vi "Fetch Class Parents Info.vi"(8 "error in (no error)":errorcluster, 11 "LVClassLibrary in":refnum<vi>) -> (0 "error out":errorcluster, 1 "Parent Interfaces":refnum<vi>[](array[refnum]), 2 "Parent Class Info":T1[](array[typedef]), 3 "LVClassLibrary out":refnum<vi>)   [LabVIEW 2023, in "VIDoc Parsing.lvlib"]
uses:
  VIDoc Parsing.lvlib
  TypeDefs/Base Class Info Cluster.ctl
  <vilib>/picture/picture.llb/imagedata.ctl
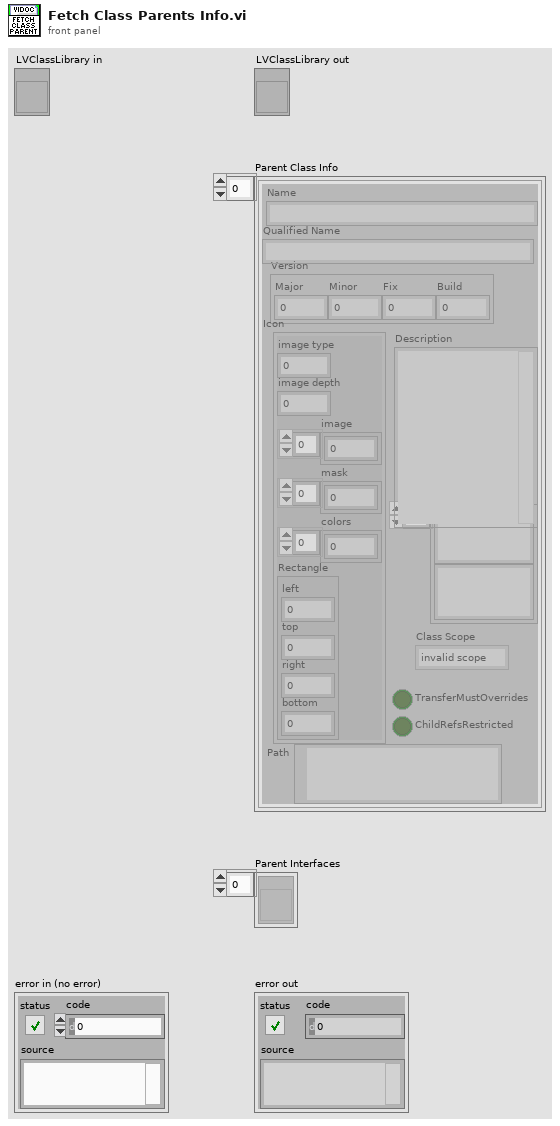
[diagram p1: front panel]
types:
  T1 = typedef "VIDoc Parsing.lvlib/Base Class Info Cluster.ctl" = cluster{"Name":string, "Icon":T2, "Version":cluster{"Major":u16, "Minor":u16, "Fix":u16, "Build":u16}, "Description":string, "Friends":string[], "ChildRefsRestricted":bool, "TransferMustOverrides":bool, "Path":path, "Qualified Name":string, "Class Scope":enum32{"invalid scope", "public", "private", "protected", "community"}}
  T2 = typedef "imagedata.ctl" = cluster{"image type":i32, "image depth":i32, "image":u8[], "mask":u8[], "colors":u32[], "Rectangle":cluster{"left":i16, "top":i16, "right":i16, "bottom":i16}}
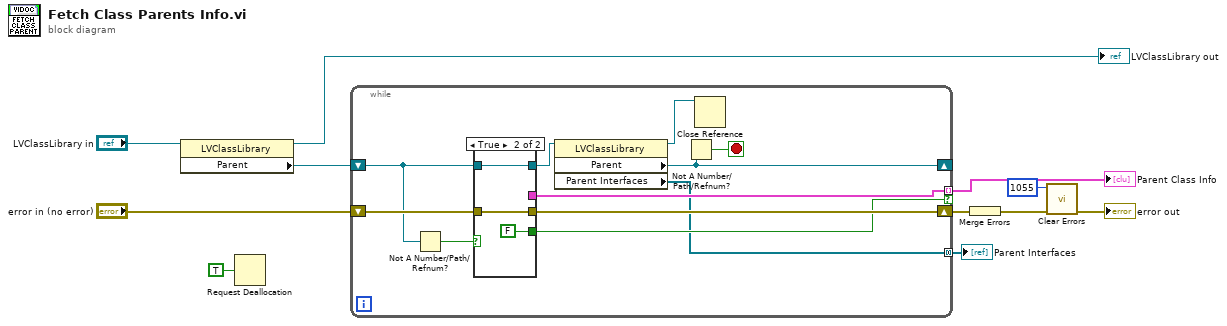
[diagram p0: block diagram]
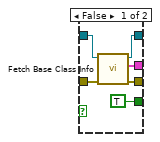
[diagram p2: hidden frame]
diagram:
  n1 = property class="LVClassLibrary"(reference="LVClassLibrary in") -> (reference out=→"LVClassLibrary out":refnum<vi>, "Parent"=w2:refnum<vi>)  [unwired: 1 in, 1 out]
  n2 = Request Deallocation(TRUE ("flag")) -> ()
  n3 = while {
    shift-right: [w18] -> _
    shift-left: w2 -> [w16]
    tunnel: [w17] -> w8 mode=indexing if=w14
    shift-right: [w20] -> w9
    shift-left: "error in (no error)" -> [w21]
    tunnel: [w13] -> w3 mode=concatenating
    stop <- w22 stop-if-true
    n4 = Not A Number/Path/Refnum?(number/path/refnum=w16) -> (NaN/Path/Refnum?=w15:bool)
    n5 = case shown="True" w15 {
      tunnel: w21 -> [w28 w30]
      tunnel: [w27 w30] -> w20
      tunnel: [w26 w31] -> w19
      tunnel: [w25 _] -> w17
      tunnel: w16 -> [w24 w31]
      tunnel: [TRUE FALSE] -> w14
      frame False {
        n6 = call "Fetch Base Class Info.vi"("error in (no error)"=w28, "LVClassLibrary in"=w24) -> ("error out"=w27:errorcluster, "Base Class Info"=w25:T1, "LVClassLibrary out"=w26:refnum<vi>)  [unwired: 7 in]
      }
      frame True {
      }
    }
    n7 = property class="LVClassLibrary"(reference=w19) -> (reference out=w12:refnum<vi>, "Parent"=w18:refnum<vi>, "Parent Interfaces"=w13:refnum<vi>[])  [unwired: 1 in, 1 out]
    n8 = Not A Number/Path/Refnum?(number/path/refnum=w18) -> (NaN/Path/Refnum?=w22:bool)
    n9 = Close Reference(reference=w12) -> ()  [unwired: 1 in, 1 out]
  }
  "Parent Class Info" <- w8
  "Parent Interfaces" <- w3
  n10 = Merge Errors(w9) -> (w7:errorcluster)
  n11 = call <vilib>:"Clear Errors.vi"("error in (no error)"=w7, "specific error code to clear (0: all)"=1055) -> ("error out"=→"error out":errorcluster)  [unwired: 4 in, 1 out]
